vi "ApplyScaleData.vi"(8 "error in (no error)":errorcluster, 10 "Image Dst":T1, 11 "Image Src":T1) -> (0 "error out":errorcluster, 3 "Corrected Image":T1(plugin-control))   [LabVIEW 2017]
uses:
  <vilib>/vision/Image Controls.llb/IMAQ Image.ctl
  <vilib>/vision/NI_Vision_Development_Module.lvlib
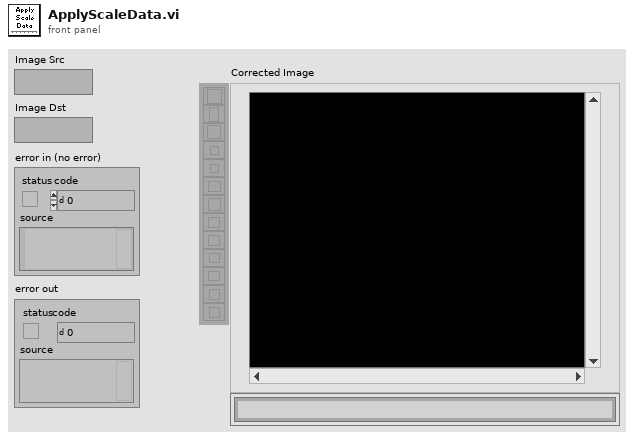
[diagram p1: front panel]
types:
  T1 = typedef "IMAQ Image.ctl" = refnum<image>
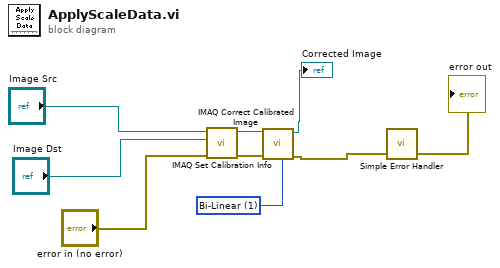
[diagram p0: block diagram]
diagram:
  w5 = u32 1 items=["Zero Order", "Bi-Linear", "Quadratic", "Cubic Spline"] ("Interpolation Type")
  n1 = call "IMAQ Set Calibration Info"("error in (no error)"="error in (no error)", "Image Dst"="Image Dst", "Image Src"="Image Src") -> ("error out"=w6:errorcluster, "Calibrated Image"=w8:T1)  [unwired: 7 in]
  n2 = call "IMAQ Correct Calibrated Image"("Interpolation Type"=w5, "error in (no error)"=w6, "Image Src"=w8) -> ("error out"=w1:errorcluster, "Corrected Image"=→"Corrected Image":T1)  [unwired: 7 in]
  "error out" <- w1
  n3 = call <vilib>:"Simple Error Handler.vi"("error in (no error)"=w1) -> ()  [unwired: 4 in, 5 out]
